vi "Save_ADAM_Table_Locally.vi"   [LabVIEW 2014]
uses:
  ADAM Controls/Update_scan_value.ctl
  Anemometry/Anemometry Sub Vis/Controls/Global_mode.ctl
  Anemometry/Anemometry Sub Vis/Globals/Trav_pos_global.vi
types:
  T1 = typedef "Global_mode.ctl" = enum16{"Read Global", "Load Global From File", "Write Global to File"}
  T2 = typedef "Update_scan_value.ctl" = cluster{"Channel Name":string, "New Value":dbl}
  T3 = typedef "Ch_description_ADAM.ctl" = cluster{"Ch Name":string, "Type":T4, "Function":T5, "Ch State":T6, "Calibration type":T7, "A":dbl, "B":dbl, "C":dbl, "D":dbl, "Comments":string, "Address":T8, "String":string, "Duty":u16}
  T4 = typedef "Module_type_ADAM.ctl" = string
  T5 = typedef "Function_ADAM.ctl" = enum16{"Analogue Input", "Digital Input", "Event counter", "Event rate", "Analogue Output", "Digital Output", "Relay Output"}
  T6 = typedef "Channel_State.ctl" = enum16{"On", "Off", "Always On", "Always Off"}
  T7 = typedef "Calib_type_ADAM.ctl" = enum16{"Raw", "Bx + A", "Cx^2 + Bx + A", "Dx^3 + Cx^2 + Bx + A", "In Band", "Hi-Tec Q", "Hi-Tec M_dot", "Text"}
  T8 = typedef "Address.ctl" = cluster{"Main":i32, "Ch.":i32, "Sub":i32, "Port Name":string}
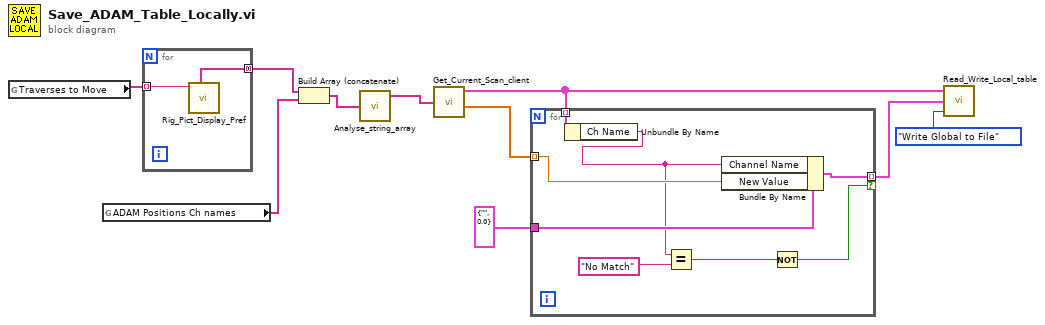
[diagram p0: block diagram]
diagram:
  n1 = global read "Trav_pos_global.vi" "Traverses to Move"() -> (w6:string[])
  n2 = global read "Trav_pos_global.vi" "ADAM Positions Ch names"() -> (w5:string[])
  n3 = for {
    tunnel: w6 -> [w12] mode=indexing
    tunnel: [w11] -> w4 mode=concatenating
    n4 = call "Rig_Pict_Display_Pref.vi"("Traverse Name"=w12) -> ("Roll Pitch Yaw ADAM Channels"=w11:string[])  [unwired: 3 in, 4 out]
  }
  n5 = Build Array (concatenate)(w4, w5) -> (w3:string[])
  n6 = call "Analyse_string_array.vi"("String array"=w3) -> ("Unique strings"=w2:string[])  [unwired: 1 in, 1 out]
  n7 = call "Get_Current_Scan_client.vi"("ADAM Ch Names"=w2) -> ("Ch Description Array"=w1:T3[], "Numerical Values"=w9:dbl[])  [unwired: 1 in, 1 out]
  n8 = for {
    tunnel: T2 {"Channel Name"="", "New Value"=0.0} ("Update Scan Value Cluster") -> [w20]
    tunnel: w9 -> [w19] mode=indexing
    tunnel: [w17] -> w7 mode=indexing if=w13
    tunnel: w1 -> [w18] mode=indexing
    n9 = Unbundle By Name(w18) -> ("Ch Name"=w15:string)
    n10 = Equal?(x=w15, y="No Match") -> (x = y?=w14:bool)
    n11 = Bundle By Name(cluster=w20, "Channel Name"=w15, "New Value"=w19) -> (w17:T2)
    n12 = Not(x=w14) -> (.not. x?=w13:bool)
  }
  n13 = call "Read_Write_Local_table.vi"("Mode"=Global_mode."Write Global to File", "Ch Values in"=w7, "Channels Descriptions In"=w1) -> ()  [unwired: 3 out]
